vi "GetChannelData.vi"(8 "error in (no error)":errorcluster, 10 "ChannelSelection":T2, 11 "reference in":refnum<k24>) -> (0 "error out":errorcluster, 1 "[Meta]Setup Info H":T1, 2 "Waveform Graph":dbl[](array[numeric]), 3 "reference out":refnum<k24>)   [LabVIEW 2019, in "LabNation Scope Driver.lvlib"]
doc: "Acquires a new set of datapoints from the scope."
uses:
  LabNation Scope Driver.lvlib
  C:/Program Files (x86)/LabNation/SmartScope/DeviceInterface.dll
  Program Files (x86)/LabNation/SmartScope/DeviceInterface.dll
  Typedef/Channel Selection.ctl
  Typedef/[Meta]Setup Info H.ctl
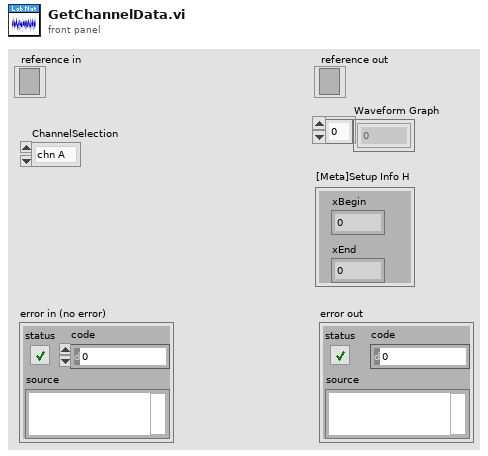
[diagram p1: front panel]
types:
  T1 = typedef "LabNation Scope Driver.lvlib/[Meta]Setup Info H.ctl" = cluster{"xBegin":dbl, "xEnd":dbl}
  T2 = typedef "LabNation Scope Driver.lvlib/Channel Selection.ctl" = enum16{"chn A", "chn B"}
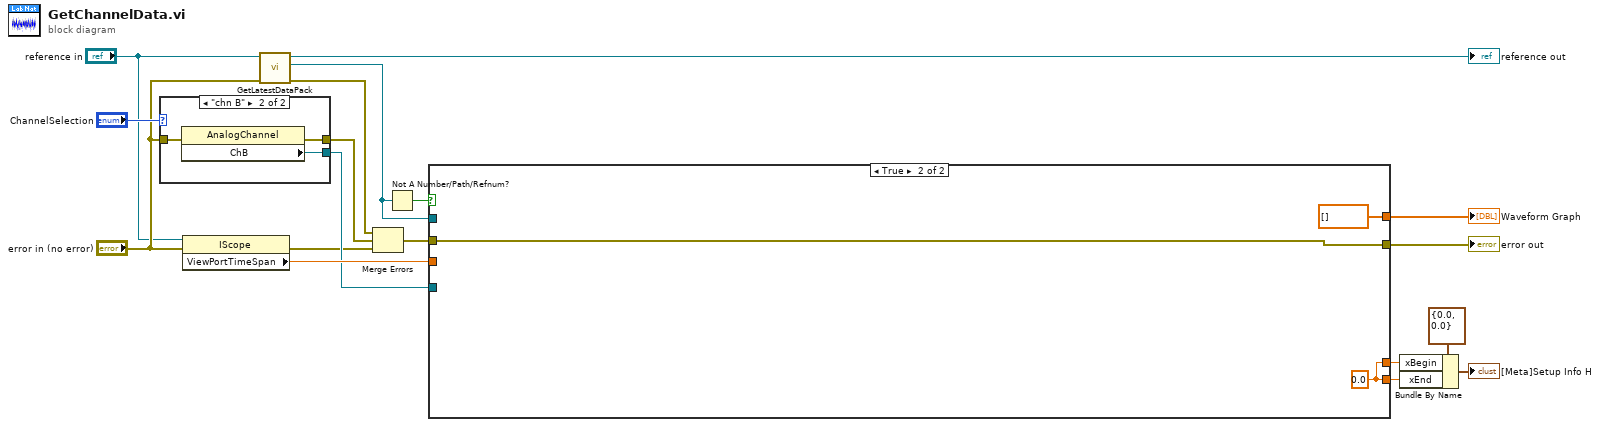
[diagram p0: block diagram]
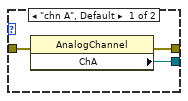
[diagram p2: hidden frame]
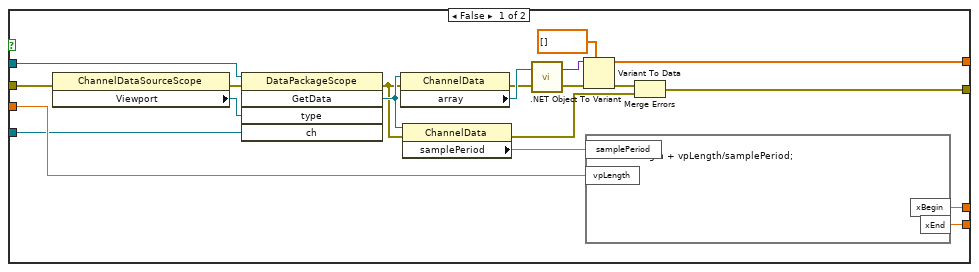
[diagram p3: hidden frame]
diagram:
  n1 = case shown="\"chn B\"" "ChannelSelection" {
    tunnel: [w21 w24] -> w13
    tunnel: [w20 w23] -> w3
    tunnel: "error in (no error)" -> [w19 w22]
    frame "chn A", Default {
      n2 = property class="AnalogChannel"(error in=w19) -> (error out=w20:errorcluster, "ChA"=w21:refnum<k24>)  [unwired: 1 in, 1 out]
    }
    frame "chn B" {
      n3 = property class="AnalogChannel"(error in=w22) -> (error out=w23:errorcluster, "ChB"=w24:refnum<k24>)  [unwired: 1 in, 1 out]
    }
  }
  n4 = property class="IScope"(reference="reference in", error in="error in (no error)") -> (error out=w11:errorcluster, "ViewPortTimeSpan"=w17:dbl)  [unwired: 1 out]
  n5 = call "GetLatestDataPack.vi"("error in (no error)"="error in (no error)", "reference in"="reference in") -> ("error out"=w4:errorcluster, "LatestDataPackage"=w16:refnum<k24>, "reference out"=→"reference out":refnum<k24>)  [unwired: 7 in]
  n6 = Merge Errors(w4, w3, w11) -> (w10:errorcluster)
  n7 = Not A Number/Path/Refnum?(number/path/refnum=w16) -> (NaN/Path/Refnum?=w18:bool)
  n8 = case shown="True" w18 {
    tunnel: w16 -> [w41 _]
    tunnel: w17 -> [w39 _]
    tunnel: [w38 dbl[] [] ("Waveform Graph")] -> w8
    tunnel: [w37 w46] -> w2
    tunnel: [w36 w46] -> w5
    tunnel: w13 -> [w35 _]
    tunnel: w10 -> [w32 w45]
    tunnel: [w26 w45] -> w9
    frame False {
      n9 = property class="ChannelDataSourceScope"(error in=w32) -> (error out=w31:errorcluster, "Viewport"=w44:refnum<k24>)  [unwired: 1 in, 1 out]
      n10 = invoke class="DataPackageScope" method="GetData"(reference=w41, error in=w31, "type"=w44, "ch"=w35) -> (error out=w25:errorcluster, "GetData"=w42:refnum<k24>)  [unwired: 1 in, 3 out]
      n11 = property class="ChannelData"(reference=w42, error in=w25) -> (error out=w30:errorcluster, "array"=w34:refnum<k24>)  [unwired: 1 out]
      n12 = property class="ChannelData"(reference=w42, error in=w25) -> (error out=w27:errorcluster, "samplePeriod"=w40:dbl)  [unwired: 1 out]
      n13 = call <vilib>:".NET Object To Variant.vi"("error in (no error)"=w30, ".NET object"=w34) -> ("error out"=w29:errorcluster, "variant"=w33:variant)
      n14 = Variant To Data(error in=w29, type=dbl[] [] ("Waveform Graph"), Variant=w33) -> (data=w38:dbl[], error out=w28:errorcluster)
      n15 = formula code="xBegin = 0;\nxEnd = xBegin + vpLength/samplePeriod;"("samplePeriod"=w40, "vpLength"=w39) -> ("xBegin"=w37:dbl, "xEnd"=w36:dbl)
      n16 = Merge Errors(w28, w27) -> (w26:errorcluster)
    }
    frame True {
      w46 = 0.0 ("xBegin")
    }
  }
  "error out" <- w9
  "Waveform Graph" <- w8
  n17 = Bundle By Name(cluster=T1 {"xBegin"=0.0, "xEnd"=0.0} ("[Meta]Setup Info H"), "xBegin"=w2, "xEnd"=w5) -> (→"[Meta]Setup Info H":T1)
